vi "validate.vi"(8 "error in":errorcluster, 11 "tag bus configurable plugin module configuration in":refnum<class "tag bus configurable plugin module configuration.lvclass">) -> (0 "error out":errorcluster, 3 "tag bus configurable plugin module configuration out":refnum<class "tag bus configurable plugin module configuration.lvclass">)   [LabVIEW 2013, in "tag bus configurable plugin module configuration.lvclass"]
doc: "This function performs validation of the configuration. This function should be safe to call at any point and should not rely on anything in the runtime environment."
uses:
  tag bus configurable plugin module configuration.lvclass
  <vilib>/NI/Tag Bus Module Framework/module configuration/TBM module configuration.lvclass
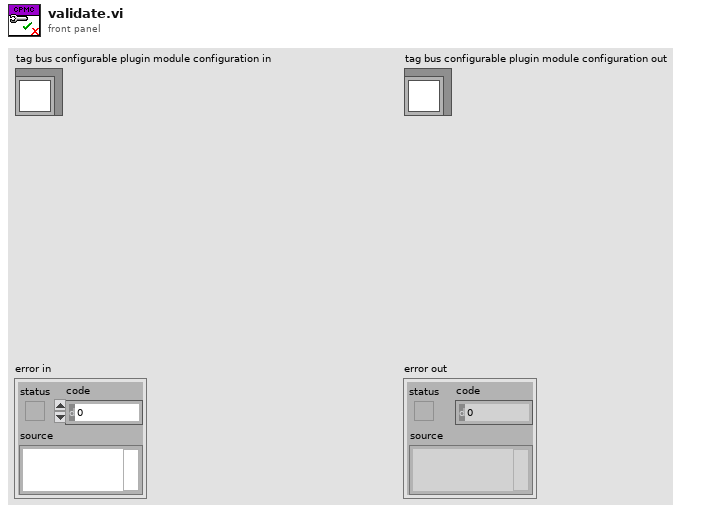
[diagram p1: front panel]
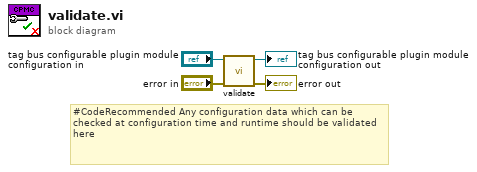
[diagram p0: block diagram]
diagram:
  # "#CodeRecommended Any configuration data which can be checked at configuration time and runtime should be validated here"
  n1 = call-parent "validate.vi"("error in"="error in", "configuration in"="tag bus configurable plugin module configuration in") -> ("error out"=→"error out":errorcluster, "configuration out"=→"tag bus configurable plugin module configuration out":refnum<class "tag bus configurable plugin module configuration.lvclass">)  [unwired: 8 in]
